vi "main.vi"() -> ()   [LabVIEW 2024]
uses:
  Global.vi
  <vilib>/Instr/_visa.llb/VISA Configure Serial Port (Instr).vi
panel:
  in  "COM-Port":refnum<visa-resource-name>
  out "Status":string
  in  "Run":bool
  in  "Remove Step":bool
  in  "Add Step":bool
  out "Program data":dbl[][](array[numeric])
  in  "Mode":u16(ring) items=["Free Run", "Acquire Program", "Run Program"]
  in  "Servo Control 4":dbl(slide) scale=0.0..100.0
  in  "Servo Control 3":dbl(slide) scale=80.0..175.0
  in  "Servo Control 2":dbl(slide) scale=70.0..140.0
  in  "Servo Control 1":dbl(slide) scale=0.0..160.0
  in  "stop":bool
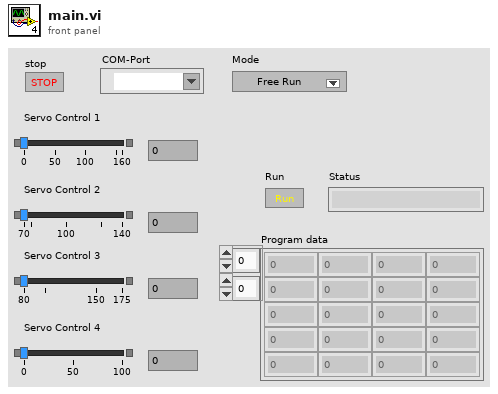
[diagram p1: front panel]
types:
  T1 = enum16{"No Change", "Serv 1", "Serv 2", "Serv 3", "Serv 4"}
  T2 = typedef "Semaphore RefNum" = refnum<k1>
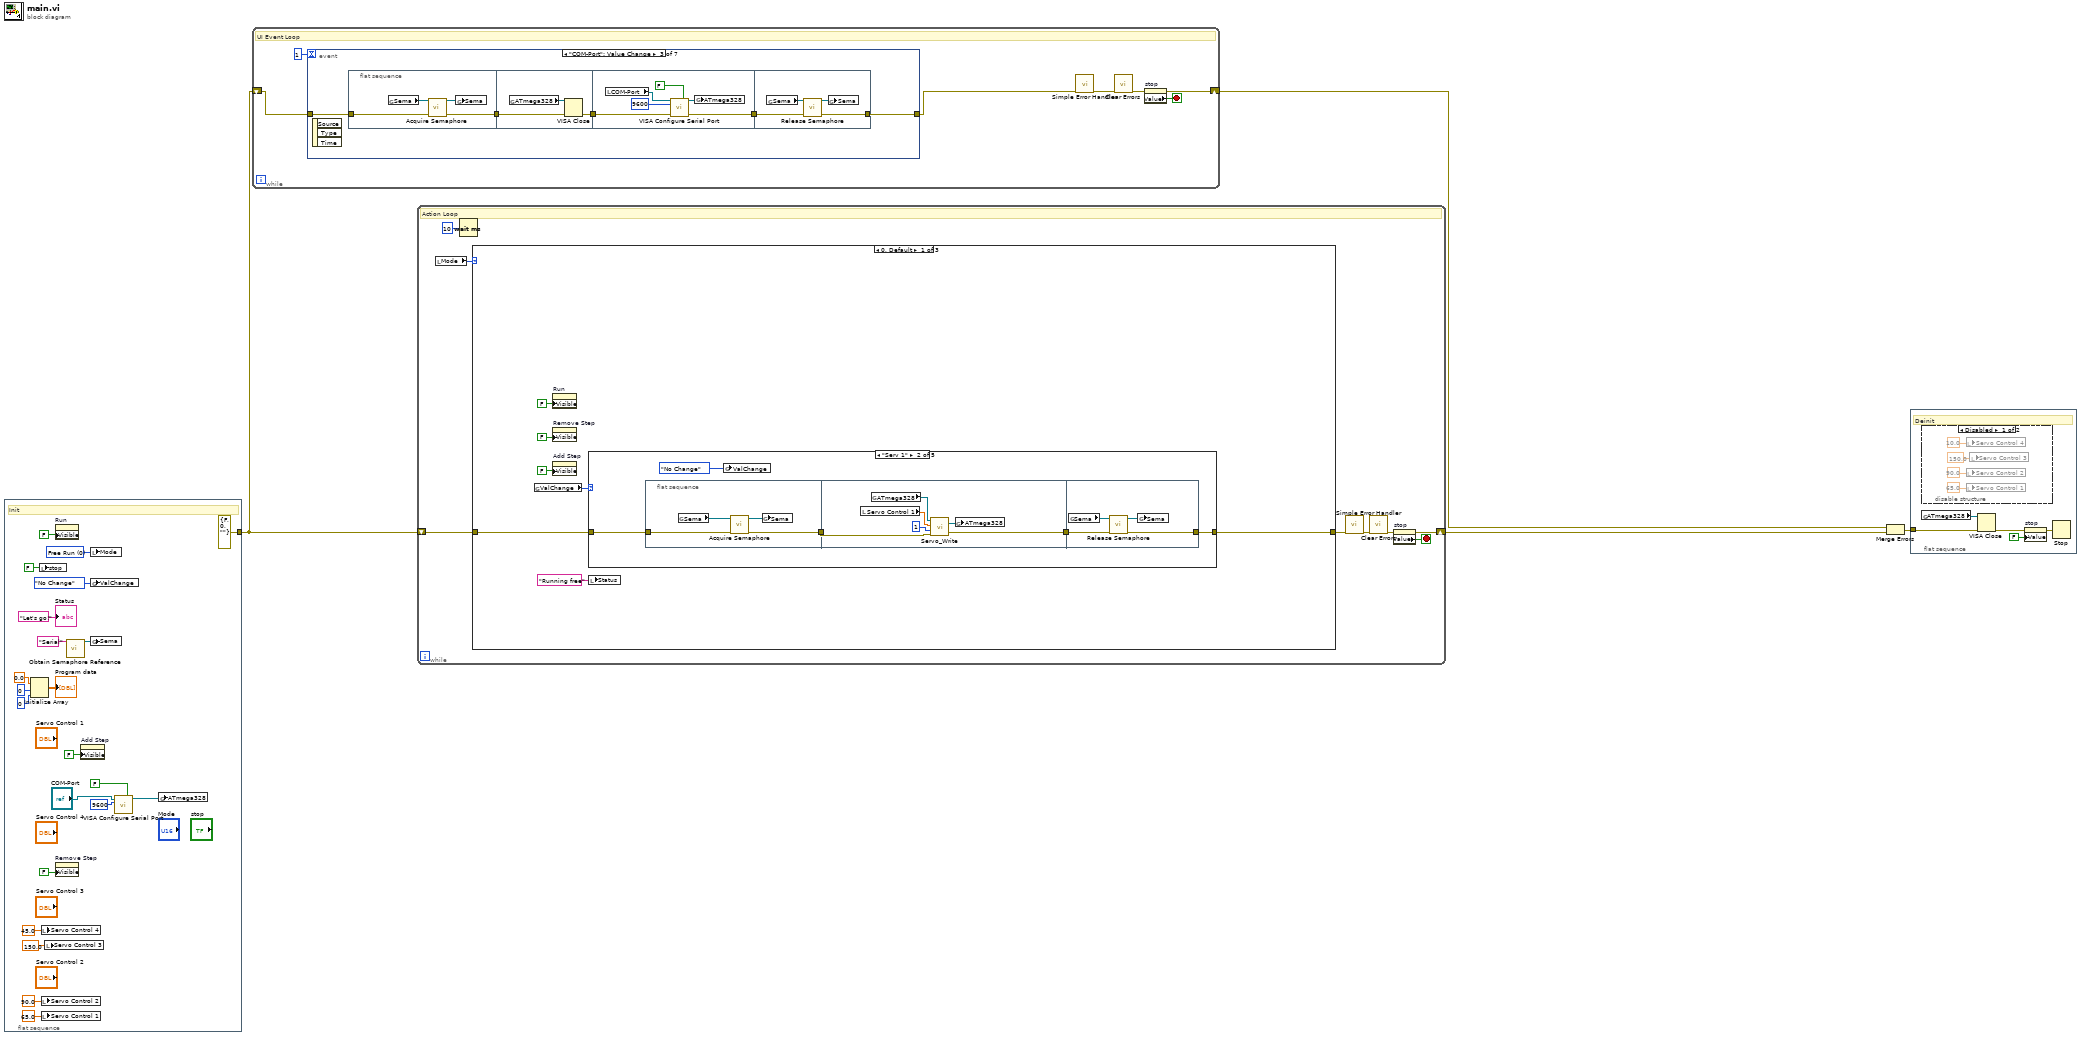
[diagram p0: block diagram]
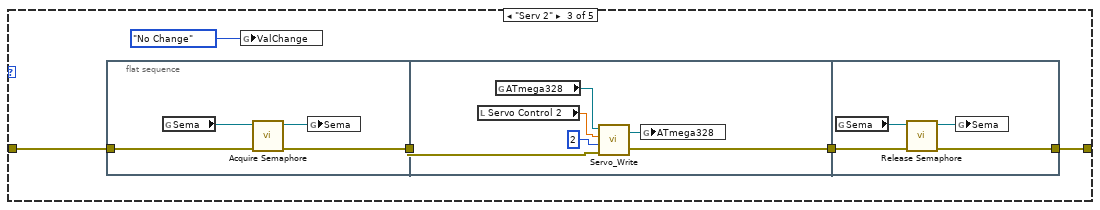
[diagram p4: hidden frame]
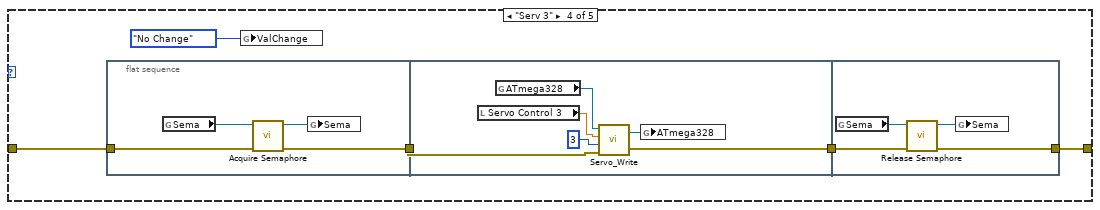
[diagram p5: hidden frame]
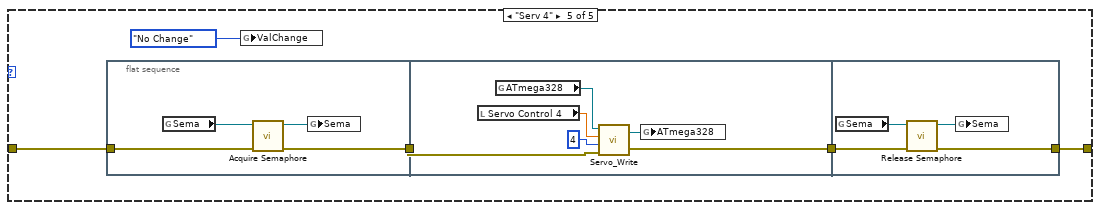
[diagram p6: hidden frame]
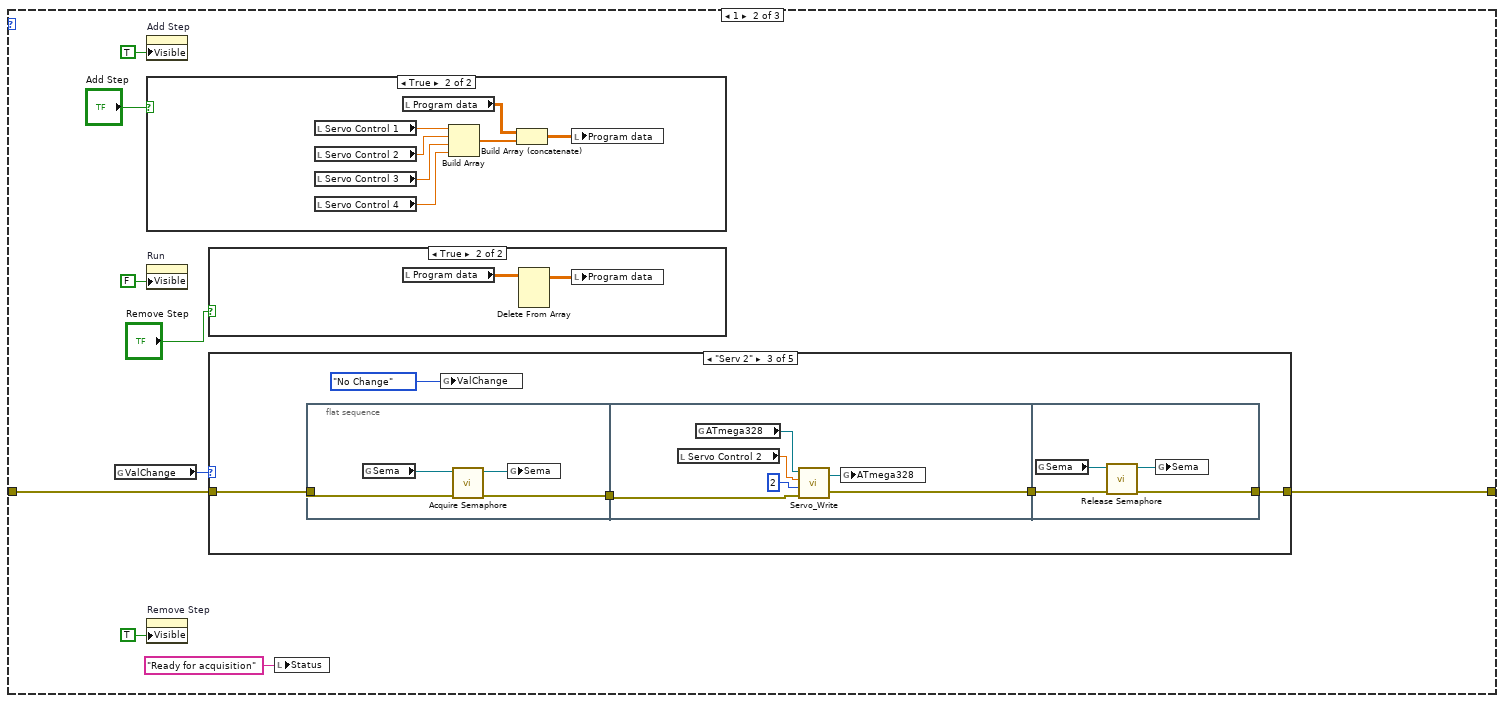
[diagram p7: hidden frame]
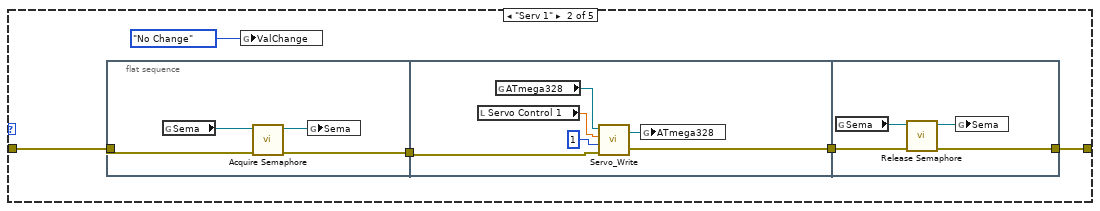
[diagram p11: hidden frame]
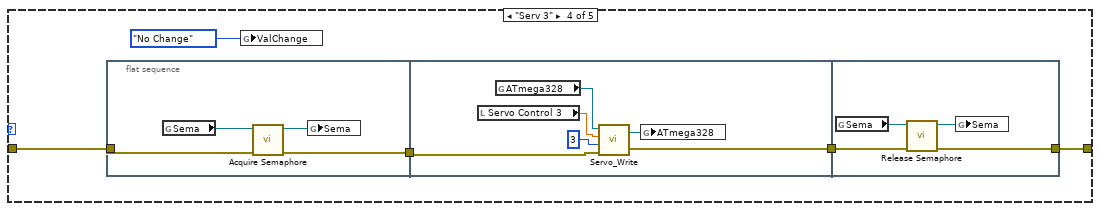
[diagram p12: hidden frame]
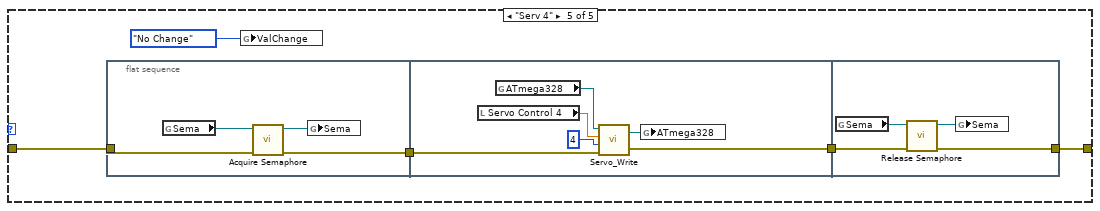
[diagram p13: hidden frame]
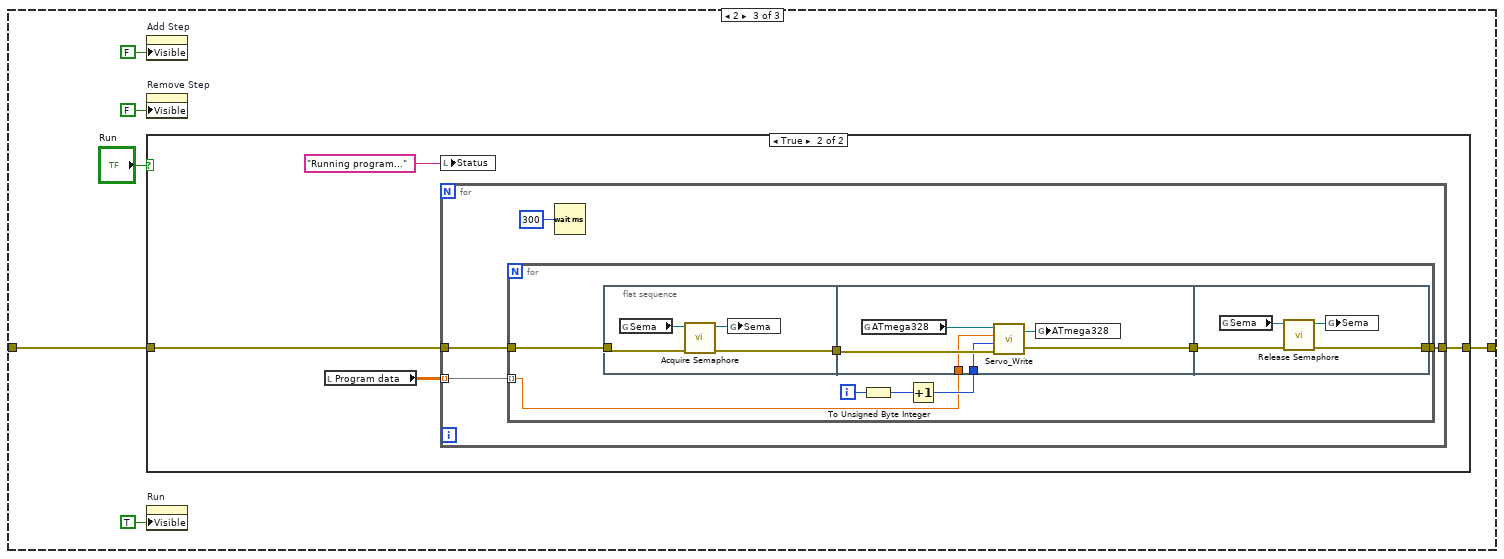
[diagram p14: hidden frame]
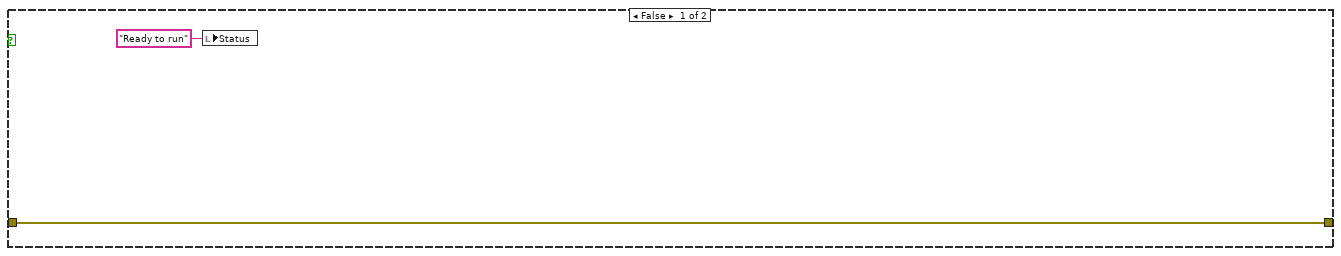
[diagram p15: hidden frame]
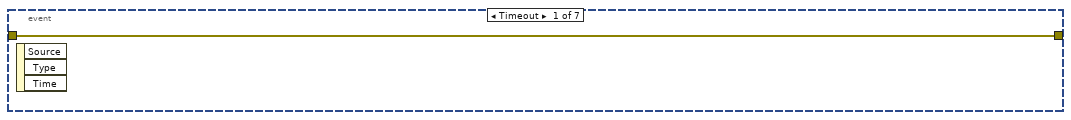
[diagram p16: hidden frame]
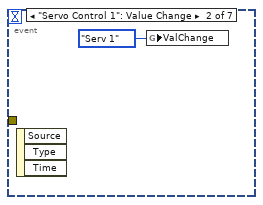
[diagram p17: hidden frame]
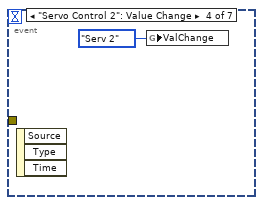
[diagram p18: hidden frame]
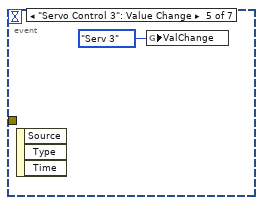
[diagram p19: hidden frame]
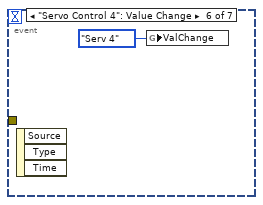
[diagram p20: hidden frame]
diagram:
  n1 = flat-sequence {
    tunnel: [errorcluster {"status"=FALSE, "code"=0, "source"=""} ("error constant")] -> w1
    frame #0 {
      w12 = u16 0 items=["Free Run", "Acquire Program", "Run Program"] ("Mode")
      # "Init"
      n2 = Initialize Array(0.0 ("element"), 0 ("dimension size"), 0 ("dimension size")) -> (→"Program data":dbl[][])
      n3 = local write "stop"(FALSE ("stop")) -> ()
      n4 = local write "Servo Control 4"(45.0 ("Servo Control 4")) -> ()
      n5 = local write "Servo Control 2"(90.0 ("Servo Control 2")) -> ()
      n6 = local write "Servo Control 1"(65.0 ("Servo Control 1")) -> ()
      n7 = local write "Servo Control 3"(150.0 ("Servo Control 3")) -> ()
      n8 = property on="Run" class="Bool"("Visible"=FALSE) -> ()  [unwired: 2 in, 2 out]
      n9 = property on="Remove Step" class="Bool"("Visible"=FALSE) -> ()  [unwired: 2 in, 2 out]
      n10 = call <vilib>:"Obtain Semaphore Reference.vi"("name (unnamed)"="Serial") -> ("semaphore"=w20:T2)  [unwired: 4 in, 2 out]
      n11 = property on="Add Step" class="Bool"("Visible"=FALSE) -> ()  [unwired: 2 in, 2 out]
      n12 = local write "Mode"(w12) -> ()
      n13 = global write "Global.vi" "ValChange"(T1."No Change" ("ValChange")) -> ()
      n14 = global write "Global.vi" "Sema"(w20) -> ()
      n15 = call-poly "VISA Configure Serial Port"("VISA resource name"="COM-Port", "Enable Termination\nChar (T)"=FALSE ("Enable Termination\nChar (T)"), "baud rate (9600)"=u32 9600) -> ("VISA resource name out"=w22:refnum<visa-resource-name>)  [unwired: 11 in, 1 out]
      n16 = global write "Global.vi" "ATmega328"(w22) -> ()
      "Status" <- "Let's go!" ("Status")
    }
  }
  n17 = while {
    shift-right: [w28] -> w4
    shift-left: w1 -> [w32]
    stop <- w33 stop-if-true
    # "UI Event Loop"
    n18 = event shown="[2] \"COM-Port\": Value Change" {
      selector: _ -> [_ _ _ _ _ _ _]
      dyn-events: _ -> [_ _ _ _ _ _ _]
      timeout: 1 -> [_ _ _ _ _ _ _]
      tunnel: [w34 _ w36 _ _ _ w61] -> w31
      tunnel: w32 -> [w34 _ w40 _ _ _ w61]
      event Timeout {
        n19 = event-data() -> ()  [unwired: 1 in, 3 out]
      }
      event "Servo Control 1": Value Change {
        n20 = event-data() -> ()  [unwired: 1 in, 3 out]
        n21 = global write "Global.vi" "ValChange"(T1."Serv 1" ("ValChange")) -> ()
      }
      event "COM-Port": Value Change {
        n22 = event-data() -> ()  [unwired: 1 in, 3 out]
        n23 = flat-sequence {
          tunnel: w40 -> [w42]
          tunnel: [w41] -> w38
          tunnel: [w45] -> w39
          tunnel: w38 -> [w46]
          tunnel: w39 -> [w50]
          tunnel: [w49] -> w37
          tunnel: w37 -> [w55]
          tunnel: [w54] -> w36
          frame #0 {
            n24 = global read "Global.vi" "Sema"() -> (w44:T2)
            n25 = call <vilib>:"Acquire Semaphore.vi"("error in (no error)"=w42, "semaphore"=w44) -> ("error out"=w41:errorcluster, "semaphore out"=w43:T2)  [unwired: 3 in, 1 out]
            n26 = global write "Global.vi" "Sema"(w43) -> ()
          }
          frame #1 {
            n27 = global read "Global.vi" "ATmega328"() -> (w47:refnum<visa-resource-name>)
            n28 = VISA Close(VISA resource name=w47, error in (no error)=w46) -> (error out=w45:errorcluster)
          }
          frame #2 {
            n29 = local read "COM-Port"() -> (w48:refnum<visa-resource-name>)
            n30 = call-poly "VISA Configure Serial Port"("VISA resource name"=w48, "Enable Termination\nChar (T)"=FALSE ("Enable Termination\nChar (T)"), "baud rate (9600)"=u32 9600, "error in (no error)"=w50) -> ("VISA resource name out"=w51:refnum<visa-resource-name>, "error out"=w49:errorcluster)  [unwired: 10 in]
            n31 = global write "Global.vi" "ATmega328"(w51) -> ()
          }
          frame #3 {
            n32 = global read "Global.vi" "Sema"() -> (w57:T2)
            n33 = call <vilib>:"Release Semaphore.vi"("error in (no error)"=w55, "semaphore"=w57) -> ("error out"=w54:errorcluster, "semaphore out"=w56:T2)  [unwired: 4 in]
            n34 = global write "Global.vi" "Sema"(w56) -> ()
          }
        }
      }
      event "Servo Control 2": Value Change {
        n35 = event-data() -> ()  [unwired: 1 in, 3 out]
        n36 = global write "Global.vi" "ValChange"(T1."Serv 2" ("ValChange")) -> ()
      }
      event "Servo Control 3": Value Change {
        n37 = event-data() -> ()  [unwired: 1 in, 3 out]
        n38 = global write "Global.vi" "ValChange"(T1."Serv 3" ("ValChange")) -> ()
      }
      event "Servo Control 4": Value Change {
        n39 = event-data() -> ()  [unwired: 1 in, 3 out]
        n40 = global write "Global.vi" "ValChange"(T1."Serv 4" ("ValChange")) -> ()
      }
      event Panel Close? {
        n41 = event-data() -> ()  [unwired: 1 in, 3 out]
        n42 = property on="stop" class="Bool (strict)"("Value"=TRUE ("stop")) -> ()  [unwired: 2 in, 2 out]
        n43 = event-data("Discard?"=FALSE) -> ()  [unwired: 1 in, 1 out]
      }
    }
    n44 = call <vilib>:"Simple Error Handler.vi"("error in (no error)"=w31) -> ("error out"=w30:errorcluster)  [unwired: 4 in, 4 out]
    n45 = call <vilib>:"Clear Errors.vi"("error in (no error)"=w30) -> ("error out"=w29:errorcluster)  [unwired: 5 in, 1 out]
    n46 = property on="stop" class="Bool (strict)"(error in=w29) -> (error out=w28:errorcluster, "Value"=w33:bool)  [unwired: 1 in, 1 out]
  }
  n47 = while {
    shift-right: [w68] -> w3
    shift-left: w1 -> [w66]
    stop <- w71 stop-if-true
    # "Action Loop"
    n48 = local read "Mode"() -> (w65:u16)
    n49 = Wait (ms)(milliseconds to wait=u32 10) -> ()  [unwired: 1 out]
    n50 = case shown="0, Default" w65 {
      tunnel: w66 -> [w77 w163 w256]
      tunnel: [w76 w160 w254] -> w64
      frame 0, Default {
        n51 = global read "Global.vi" "ValChange"() -> (w78:T1)
        n52 = property on="Run" class="Bool"("Visible"=FALSE) -> ()  [unwired: 2 in, 2 out]
        n53 = property on="Remove Step" class="Bool"("Visible"=FALSE) -> ()  [unwired: 2 in, 2 out]
        n54 = property on="Add Step" class="Bool"("Visible"=FALSE) -> ()  [unwired: 2 in, 2 out]
        n55 = case shown="\"Serv 1\"" w78 {
          tunnel: w77 -> [w79 w84 w103 w122 w141]
          tunnel: [w79 w81 w100 w119 w138] -> w76
          frame "No Change", Default {
          }
          frame "Serv 1" {
            n56 = flat-sequence {
              tunnel: w84 -> [w86]
              tunnel: [w85] -> w83
              tunnel: w83 -> [w92]
              tunnel: [w91] -> w82
              tunnel: w82 -> [w96]
              tunnel: [w95] -> w81
              frame #0 {
                n57 = global read "Global.vi" "Sema"() -> (w88:T2)
                n58 = call <vilib>:"Acquire Semaphore.vi"("error in (no error)"=w86, "semaphore"=w88) -> ("error out"=w85:errorcluster, "semaphore out"=w87:T2)  [unwired: 3 in, 1 out]
                n59 = global write "Global.vi" "Sema"(w87) -> ()
              }
              frame #1 {
                n60 = local read "Servo Control 1"() -> (w90:dbl)
                n61 = global read "Global.vi" "ATmega328"() -> (w94:refnum<visa-resource-name>)
                n62 = call "Servo_Write.vi"("error in (no error)"=w92, "Servo Index"=u8 1, "Servo Control"=w90, "VISA resource name"=w94) -> ("error out"=w91:errorcluster, "VISA resource name out"=w93:refnum<visa-resource-name>)
                n63 = global write "Global.vi" "ATmega328"(w93) -> ()
              }
              frame #2 {
                n64 = global read "Global.vi" "Sema"() -> (w98:T2)
                n65 = call <vilib>:"Release Semaphore.vi"("error in (no error)"=w96, "semaphore"=w98) -> ("error out"=w95:errorcluster, "semaphore out"=w97:T2)  [unwired: 4 in]
                n66 = global write "Global.vi" "Sema"(w97) -> ()
              }
            }
            n67 = global write "Global.vi" "ValChange"(T1."No Change" ("ValChange")) -> ()
          }
          frame "Serv 2" {
            n68 = flat-sequence {
              tunnel: w103 -> [w105]
              tunnel: [w104] -> w102
              tunnel: w102 -> [w111]
              tunnel: [w110] -> w101
              tunnel: w101 -> [w115]
              tunnel: [w114] -> w100
              frame #0 {
                n69 = global read "Global.vi" "Sema"() -> (w107:T2)
                n70 = call <vilib>:"Acquire Semaphore.vi"("error in (no error)"=w105, "semaphore"=w107) -> ("error out"=w104:errorcluster, "semaphore out"=w106:T2)  [unwired: 3 in, 1 out]
                n71 = global write "Global.vi" "Sema"(w106) -> ()
              }
              frame #1 {
                n72 = local read "Servo Control 2"() -> (w109:dbl)
                n73 = global read "Global.vi" "ATmega328"() -> (w113:refnum<visa-resource-name>)
                n74 = call "Servo_Write.vi"("error in (no error)"=w111, "Servo Index"=u8 2, "Servo Control"=w109, "VISA resource name"=w113) -> ("error out"=w110:errorcluster, "VISA resource name out"=w112:refnum<visa-resource-name>)
                n75 = global write "Global.vi" "ATmega328"(w112) -> ()
              }
              frame #2 {
                n76 = global read "Global.vi" "Sema"() -> (w117:T2)
                n77 = call <vilib>:"Release Semaphore.vi"("error in (no error)"=w115, "semaphore"=w117) -> ("error out"=w114:errorcluster, "semaphore out"=w116:T2)  [unwired: 4 in]
                n78 = global write "Global.vi" "Sema"(w116) -> ()
              }
            }
            n79 = global write "Global.vi" "ValChange"(T1."No Change" ("ValChange")) -> ()
          }
          frame "Serv 3" {
            n80 = flat-sequence {
              tunnel: w122 -> [w124]
              tunnel: [w123] -> w121
              tunnel: w121 -> [w130]
              tunnel: [w129] -> w120
              tunnel: w120 -> [w134]
              tunnel: [w133] -> w119
              frame #0 {
                n81 = global read "Global.vi" "Sema"() -> (w126:T2)
                n82 = call <vilib>:"Acquire Semaphore.vi"("error in (no error)"=w124, "semaphore"=w126) -> ("error out"=w123:errorcluster, "semaphore out"=w125:T2)  [unwired: 3 in, 1 out]
                n83 = global write "Global.vi" "Sema"(w125) -> ()
              }
              frame #1 {
                n84 = local read "Servo Control 3"() -> (w128:dbl)
                n85 = global read "Global.vi" "ATmega328"() -> (w132:refnum<visa-resource-name>)
                n86 = call "Servo_Write.vi"("error in (no error)"=w130, "Servo Index"=u8 3, "Servo Control"=w128, "VISA resource name"=w132) -> ("error out"=w129:errorcluster, "VISA resource name out"=w131:refnum<visa-resource-name>)
                n87 = global write "Global.vi" "ATmega328"(w131) -> ()
              }
              frame #2 {
                n88 = global read "Global.vi" "Sema"() -> (w136:T2)
                n89 = call <vilib>:"Release Semaphore.vi"("error in (no error)"=w134, "semaphore"=w136) -> ("error out"=w133:errorcluster, "semaphore out"=w135:T2)  [unwired: 4 in]
                n90 = global write "Global.vi" "Sema"(w135) -> ()
              }
            }
            n91 = global write "Global.vi" "ValChange"(T1."No Change" ("ValChange")) -> ()
          }
          frame "Serv 4" {
            n92 = flat-sequence {
              tunnel: w141 -> [w143]
              tunnel: [w142] -> w140
              tunnel: w140 -> [w149]
              tunnel: [w148] -> w139
              tunnel: w139 -> [w153]
              tunnel: [w152] -> w138
              frame #0 {
                n93 = global read "Global.vi" "Sema"() -> (w145:T2)
                n94 = call <vilib>:"Acquire Semaphore.vi"("error in (no error)"=w143, "semaphore"=w145) -> ("error out"=w142:errorcluster, "semaphore out"=w144:T2)  [unwired: 3 in, 1 out]
                n95 = global write "Global.vi" "Sema"(w144) -> ()
              }
              frame #1 {
                n96 = local read "Servo Control 4"() -> (w146:dbl)
                n97 = global read "Global.vi" "ATmega328"() -> (w151:refnum<visa-resource-name>)
                n98 = call "Servo_Write.vi"("error in (no error)"=w149, "Servo Index"=u8 4, "Servo Control"=w146, "VISA resource name"=w151) -> ("error out"=w148:errorcluster, "VISA resource name out"=w150:refnum<visa-resource-name>)
                n99 = global write "Global.vi" "ATmega328"(w150) -> ()
              }
              frame #2 {
                n100 = global read "Global.vi" "Sema"() -> (w155:T2)
                n101 = call <vilib>:"Release Semaphore.vi"("error in (no error)"=w153, "semaphore"=w155) -> ("error out"=w152:errorcluster, "semaphore out"=w154:T2)  [unwired: 4 in]
                n102 = global write "Global.vi" "Sema"(w154) -> ()
              }
            }
            n103 = global write "Global.vi" "ValChange"(T1."No Change" ("ValChange")) -> ()
          }
        }
        n104 = local write "Status"("Running free" ("Status")) -> ()
      }
      frame 1 {
        n105 = global read "Global.vi" "ValChange"() -> (w164:T1)
        n106 = property on="Add Step" class="Bool"("Visible"=TRUE) -> ()  [unwired: 2 in, 2 out]
        n107 = case shown="True" "Add Step" {
          frame False {
          }
          frame True {
            n108 = local read "Servo Control 1"() -> (w173:dbl)
            n109 = local read "Servo Control 2"() -> (w172:dbl)
            n110 = local read "Servo Control 3"() -> (w171:dbl)
            n111 = local read "Servo Control 4"() -> (w170:dbl)
            n112 = local read "Program data"() -> (w169:dbl[][])
            n113 = Build Array(w173, w172, w171, w170) -> (w168:dbl[])
            n114 = Build Array (concatenate)(w169, w168) -> (w167:dbl[][])
            n115 = local write "Program data"(w167) -> ()
          }
        }
        n116 = property on="Run" class="Bool"("Visible"=FALSE) -> ()  [unwired: 2 in, 2 out]
        n117 = property on="Remove Step" class="Bool"("Visible"=TRUE) -> ()  [unwired: 2 in, 2 out]
        n118 = case shown="True" "Remove Step" {
          frame False {
          }
          frame True {
            n119 = local read "Program data"() -> (w166:dbl[][])
            n120 = Delete From Array(array=w166) -> (array with subset deleted=w165:dbl[][])  [unwired: 3 in, 1 out]
            n121 = local write "Program data"(w165) -> ()
          }
        }
        n122 = case shown="\"Serv 2\"" w164 {
          tunnel: w163 -> [w174 w179 w198 w217 w236]
          tunnel: [w174 w176 w195 w214 w233] -> w160
          frame "No Change", Default {
          }
          frame "Serv 1" {
            n123 = flat-sequence {
              tunnel: w179 -> [w181]
              tunnel: [w180] -> w178
              tunnel: w178 -> [w187]
              tunnel: [w186] -> w177
              tunnel: w177 -> [w191]
              tunnel: [w190] -> w176
              frame #0 {
                n124 = global read "Global.vi" "Sema"() -> (w183:T2)
                n125 = call <vilib>:"Acquire Semaphore.vi"("error in (no error)"=w181, "semaphore"=w183) -> ("error out"=w180:errorcluster, "semaphore out"=w182:T2)  [unwired: 3 in, 1 out]
                n126 = global write "Global.vi" "Sema"(w182) -> ()
              }
              frame #1 {
                n127 = local read "Servo Control 1"() -> (w185:dbl)
                n128 = global read "Global.vi" "ATmega328"() -> (w189:refnum<visa-resource-name>)
                n129 = call "Servo_Write.vi"("error in (no error)"=w187, "Servo Index"=u8 1, "Servo Control"=w185, "VISA resource name"=w189) -> ("error out"=w186:errorcluster, "VISA resource name out"=w188:refnum<visa-resource-name>)
                n130 = global write "Global.vi" "ATmega328"(w188) -> ()
              }
              frame #2 {
                n131 = global read "Global.vi" "Sema"() -> (w193:T2)
                n132 = call <vilib>:"Release Semaphore.vi"("error in (no error)"=w191, "semaphore"=w193) -> ("error out"=w190:errorcluster, "semaphore out"=w192:T2)  [unwired: 4 in]
                n133 = global write "Global.vi" "Sema"(w192) -> ()
              }
            }
            n134 = global write "Global.vi" "ValChange"(T1."No Change" ("ValChange")) -> ()
          }
          frame "Serv 2" {
            n135 = flat-sequence {
              tunnel: w198 -> [w200]
              tunnel: [w199] -> w197
              tunnel: w197 -> [w206]
              tunnel: [w205] -> w196
              tunnel: w196 -> [w210]
              tunnel: [w209] -> w195
              frame #0 {
                n136 = global read "Global.vi" "Sema"() -> (w202:T2)
                n137 = call <vilib>:"Acquire Semaphore.vi"("error in (no error)"=w200, "semaphore"=w202) -> ("error out"=w199:errorcluster, "semaphore out"=w201:T2)  [unwired: 3 in, 1 out]
                n138 = global write "Global.vi" "Sema"(w201) -> ()
              }
              frame #1 {
                n139 = local read "Servo Control 2"() -> (w204:dbl)
                n140 = global read "Global.vi" "ATmega328"() -> (w208:refnum<visa-resource-name>)
                n141 = call "Servo_Write.vi"("error in (no error)"=w206, "Servo Index"=u8 2, "Servo Control"=w204, "VISA resource name"=w208) -> ("error out"=w205:errorcluster, "VISA resource name out"=w207:refnum<visa-resource-name>)
                n142 = global write "Global.vi" "ATmega328"(w207) -> ()
              }
              frame #2 {
                n143 = global read "Global.vi" "Sema"() -> (w212:T2)
                n144 = call <vilib>:"Release Semaphore.vi"("error in (no error)"=w210, "semaphore"=w212) -> ("error out"=w209:errorcluster, "semaphore out"=w211:T2)  [unwired: 4 in]
                n145 = global write "Global.vi" "Sema"(w211) -> ()
              }
            }
            n146 = global write "Global.vi" "ValChange"(T1."No Change" ("ValChange")) -> ()
          }
          frame "Serv 3" {
            n147 = flat-sequence {
              tunnel: w217 -> [w219]
              tunnel: [w218] -> w216
              tunnel: w216 -> [w225]
              tunnel: [w224] -> w215
              tunnel: w215 -> [w229]
              tunnel: [w228] -> w214
              frame #0 {
                n148 = global read "Global.vi" "Sema"() -> (w221:T2)
                n149 = call <vilib>:"Acquire Semaphore.vi"("error in (no error)"=w219, "semaphore"=w221) -> ("error out"=w218:errorcluster, "semaphore out"=w220:T2)  [unwired: 3 in, 1 out]
                n150 = global write "Global.vi" "Sema"(w220) -> ()
              }
              frame #1 {
                n151 = local read "Servo Control 3"() -> (w223:dbl)
                n152 = global read "Global.vi" "ATmega328"() -> (w227:refnum<visa-resource-name>)
                n153 = call "Servo_Write.vi"("error in (no error)"=w225, "Servo Index"=u8 3, "Servo Control"=w223, "VISA resource name"=w227) -> ("error out"=w224:errorcluster, "VISA resource name out"=w226:refnum<visa-resource-name>)
                n154 = global write "Global.vi" "ATmega328"(w226) -> ()
              }
              frame #2 {
                n155 = global read "Global.vi" "Sema"() -> (w231:T2)
                n156 = call <vilib>:"Release Semaphore.vi"("error in (no error)"=w229, "semaphore"=w231) -> ("error out"=w228:errorcluster, "semaphore out"=w230:T2)  [unwired: 4 in]
                n157 = global write "Global.vi" "Sema"(w230) -> ()
              }
            }
            n158 = global write "Global.vi" "ValChange"(T1."No Change" ("ValChange")) -> ()
          }
          frame "Serv 4" {
            n159 = flat-sequence {
              tunnel: w236 -> [w238]
              tunnel: [w237] -> w235
              tunnel: w235 -> [w244]
              tunnel: [w243] -> w234
              tunnel: w234 -> [w248]
              tunnel: [w247] -> w233
              frame #0 {
                n160 = global read "Global.vi" "Sema"() -> (w240:T2)
                n161 = call <vilib>:"Acquire Semaphore.vi"("error in (no error)"=w238, "semaphore"=w240) -> ("error out"=w237:errorcluster, "semaphore out"=w239:T2)  [unwired: 3 in, 1 out]
                n162 = global write "Global.vi" "Sema"(w239) -> ()
              }
              frame #1 {
                n163 = local read "Servo Control 4"() -> (w241:dbl)
                n164 = global read "Global.vi" "ATmega328"() -> (w246:refnum<visa-resource-name>)
                n165 = call "Servo_Write.vi"("error in (no error)"=w244, "Servo Index"=u8 4, "Servo Control"=w241, "VISA resource name"=w246) -> ("error out"=w243:errorcluster, "VISA resource name out"=w245:refnum<visa-resource-name>)
                n166 = global write "Global.vi" "ATmega328"(w245) -> ()
              }
              frame #2 {
                n167 = global read "Global.vi" "Sema"() -> (w250:T2)
                n168 = call <vilib>:"Release Semaphore.vi"("error in (no error)"=w248, "semaphore"=w250) -> ("error out"=w247:errorcluster, "semaphore out"=w249:T2)  [unwired: 4 in]
                n169 = global write "Global.vi" "Sema"(w249) -> ()
              }
            }
            n170 = global write "Global.vi" "ValChange"(T1."No Change" ("ValChange")) -> ()
          }
        }
        n171 = local write "Status"("Ready for acquisition" ("Status")) -> ()
      }
      frame 2 {
        n172 = property on="Add Step" class="Bool"("Visible"=FALSE) -> ()  [unwired: 2 in, 2 out]
        n173 = property on="Remove Step" class="Bool"("Visible"=FALSE) -> ()  [unwired: 2 in, 2 out]
        n174 = case shown="True" "Run" {
          tunnel: w256 -> [w258 w260]
          tunnel: [w258 w259] -> w254
          frame False {
            n175 = local write "Status"("Ready to run" ("Status")) -> ()
          }
          frame True {
            n176 = local read "Program data"() -> (w261:dbl[][])
            n177 = local write "Status"("Running program..." ("Status")) -> ()
            n178 = for {
              tunnel: w261 -> [w265] mode=indexing
              tunnel: w260 -> [w264]
              tunnel: [w263] -> w259
              n179 = for {
                tunnel: w265 -> [w270] mode=indexing
                tunnel: w264 -> [w268]
                tunnel: [w267] -> w263
                i -> [w272]
                n180 = flat-sequence {
                  tunnel: [w276] -> w274
                  tunnel: w268 -> [w275]
                  tunnel: w274 -> [w282]
                  tunnel: [w281] -> w273
                  tunnel: w271 -> [w280]
                  tunnel: w270 -> [w279]
                  tunnel: w273 -> [w286]
                  tunnel: [w285] -> w267
                  frame #0 {
                    n181 = global read "Global.vi" "Sema"() -> (w278:T2)
                    n182 = call <vilib>:"Acquire Semaphore.vi"("error in (no error)"=w275, "semaphore"=w278) -> ("error out"=w276:errorcluster, "semaphore out"=w277:T2)  [unwired: 3 in, 1 out]
                    n183 = global write "Global.vi" "Sema"(w277) -> ()
                  }
                  frame #1 {
                    n184 = global read "Global.vi" "ATmega328"() -> (w284:refnum<visa-resource-name>)
                    n185 = call "Servo_Write.vi"("error in (no error)"=w282, "Servo Index"=w280, "Servo Control"=w279, "VISA resource name"=w284) -> ("error out"=w281:errorcluster, "VISA resource name out"=w283:refnum<visa-resource-name>)
                    n186 = global write "Global.vi" "ATmega328"(w283) -> ()
                  }
                  frame #2 {
                    n187 = global read "Global.vi" "Sema"() -> (w288:T2)
                    n188 = call <vilib>:"Release Semaphore.vi"("error in (no error)"=w286, "semaphore"=w288) -> ("error out"=w285:errorcluster, "semaphore out"=w287:T2)  [unwired: 4 in]
                    n189 = global write "Global.vi" "Sema"(w287) -> ()
                  }
                }
                n190 = To Unsigned Byte Integer(number=w272) -> (unsigned 8bit integer=w269:u8)
                n191 = Increment(x=w269) -> (x+1=w271:u8)
              }
              n192 = Wait (ms)(milliseconds to wait=u32 300) -> ()  [unwired: 1 out]
            }
          }
        }
        n193 = property on="Run" class="Bool"("Visible"=TRUE) -> ()  [unwired: 2 in, 2 out]
      }
    }
    n194 = call <vilib>:"Simple Error Handler.vi"("error in (no error)"=w64) -> ("error out"=w70:errorcluster)  [unwired: 4 in, 4 out]
    n195 = call <vilib>:"Clear Errors.vi"("error in (no error)"=w70) -> ("error out"=w69:errorcluster)  [unwired: 5 in, 1 out]
    n196 = property on="stop" class="Bool (strict)"(error in=w69) -> (error out=w68:errorcluster, "Value"=w71:bool)  [unwired: 1 in, 1 out]
  }
  n197 = Merge Errors(w4, w3) -> (w2:errorcluster)
  n198 = flat-sequence {
    tunnel: w2 -> [w293]
    frame #0 {
      # "Deinit"
      n199 = disable-structure shown="Disabled" {
        frame Disabled {
          n200 = local write "Servo Control 4"(10.0 ("Servo Control 4")) -> ()
          n201 = local write "Servo Control 2"(90.0 ("Servo Control 2")) -> ()
          n202 = local write "Servo Control 1"(65.0 ("Servo Control 1")) -> ()
          n203 = local write "Servo Control 3"(150.0 ("Servo Control 3")) -> ()
        }
        frame Enabled {
        }
      }
      n204 = global read "Global.vi" "ATmega328"() -> (w292:refnum<visa-resource-name>)
      n205 = VISA Close(VISA resource name=w292, error in (no error)=w293) -> (error out=w290:errorcluster)
      n206 = property on="stop" class="Bool (strict)"(error in=w290, "Value"=FALSE ("stop")) -> (error out=w289:errorcluster)  [unwired: 1 in, 1 out]
      n207 = Stop(stop? (T)=w289) -> ()
    }
  }
